vi "array_maker2.vi"(6 "WEIGHT":dbl[](array[numeric]), 11 "Array":dbl[][](array[numeric])) -> (3 "Array 2":dbl[][](array[numeric]))   [LabVIEW 2013]
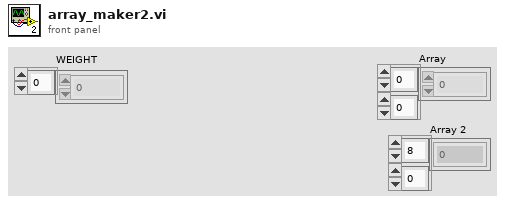
[diagram p1: front panel]
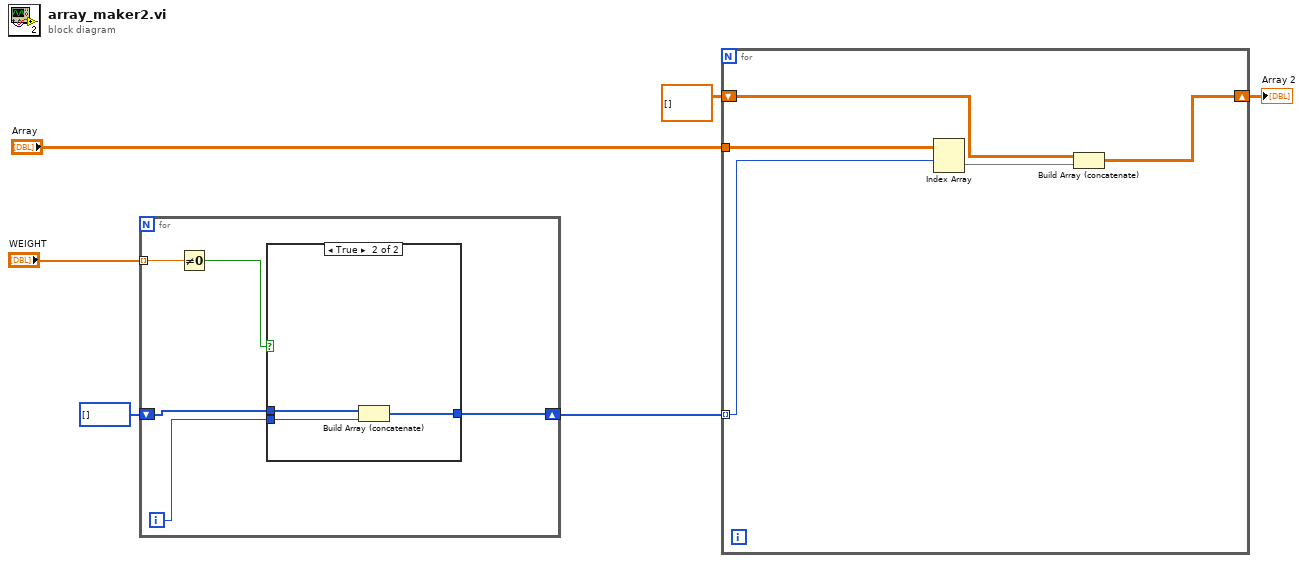
[diagram p0: block diagram]
diagram:
  n1 = for {
    tunnel: "WEIGHT" -> [w11] mode=indexing
    shift-right: [w8] -> w4
    shift-left: i32[] [] -> [w7]
    i -> [w9]
    n2 = Not Equal To 0?(x=w11) -> (x != 0?=w10:bool)
    n3 = case shown="True" w10 {
      tunnel: w9 -> [_ w15]
      tunnel: [w12 w14] -> w8
      tunnel: w7 -> [w12 w13]
      frame False {
      }
      frame True {
        n4 = Build Array (concatenate)(w13, w15) -> (w14:i32[])
      }
    }
  }
  n5 = for {
    tunnel: w4 -> [w19] mode=indexing
    tunnel: "Array" -> [w20]
    shift-right: [w17] -> w1
    shift-left: dbl[][] [] -> [w16]
    n6 = Index Array(array=w20, index (row)=w19) -> (element=w18:dbl[])  [unwired: 1 in]
    n7 = Build Array (concatenate)(w16, w18) -> (w17:dbl[][])
  }
  "Array 2" <- w1
